vi "channel.name.vi"(8 "error in":errorcluster, 11 "Channel in":refnum<class "Channel.lvclass">) -> (0 "error out":errorcluster, 3 "Channel out":refnum<class "Channel.lvclass">)   [LabVIEW 2020, in "Channel.lvclass"]
doc: "Returns the channel's name."
uses:
  Channel.lvclass
  Channel.lvclass/Channel.ctl
  client.lvlib
panel:
  out "out_needed out":u32
  out "name":string
  in  "buf":string
  in  "cap":u32
  in  "out_needed":u32
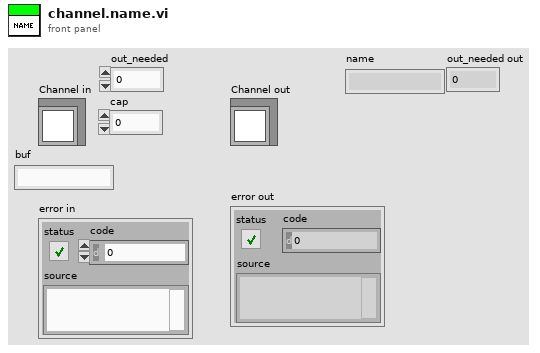
[diagram p1: front panel]
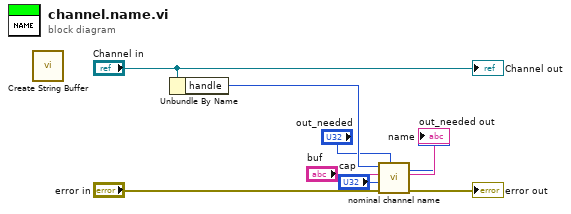
[diagram p0: block diagram]
diagram:
  n1 = call "Create String Buffer.vi"() -> ()  [unwired: 9 in, 3 out]
  n2 = Unbundle By Name("Channel in") -> ("handle"=w7:i32)
  n3 = call "nominal channel name.vi"("out_needed"="out_needed", "error in (no error)"="error in", "cap"="cap", "buf"="buf", "channel"=w7) -> ("error out"=→"error out":errorcluster, "buf out"=→"name":string, "out_needed out"=→"out_needed out":u32)  [unwired: 3 in, 1 out]
  "Channel out" <- "Channel in"
